vi "Cycle.vi"(8 "error in (no error)":errorcluster, 11 "MultDimExperiment In":refnum<class "MultDimExperiment.lvclass">) -> (0 "error out":errorcluster, 3 "MultDimExperiment Out":refnum<class "MultDimExperiment.lvclass">)   [LabVIEW 2010]
uses:
  MultDimExperiment.lvclass
panel:
  out "XY Graph":cluster{"horizontal":dbl[], "vertical":dbl[]}[](graph)
  out "ExperimentStats":T1
  in  "FixationRadius":dbl=50.0
  in  "RewardAmount":dbl=50.0
  in  "Timeouts":T2={"Intertrial"=1000.0, "AcquireFixation"=1000.0, "HoldFixation"=300.0, "DelayPeriod"=1000.0, "ResponsePeriod"=1000.0}
  in  "Eye Params":dbl[](array[numeric])
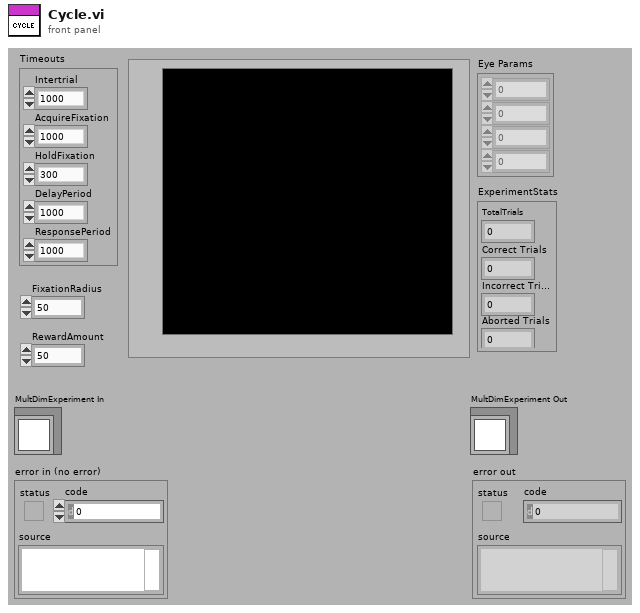
[diagram p1: front panel]
types:
  T1 = cluster{"TotalTrials":dbl, "Correct Trials":dbl, "Incorrect Trials":dbl, "Aborted Trials":dbl}
  T2 = cluster{"Intertrial":dbl, "AcquireFixation":dbl, "HoldFixation":dbl, "DelayPeriod":dbl, "ResponsePeriod":dbl}
  T3 = cluster{"TotalTrials":u32, "Correct Trials":u32, "Incorrect Trials":u32, "Aborted Trials":u32}
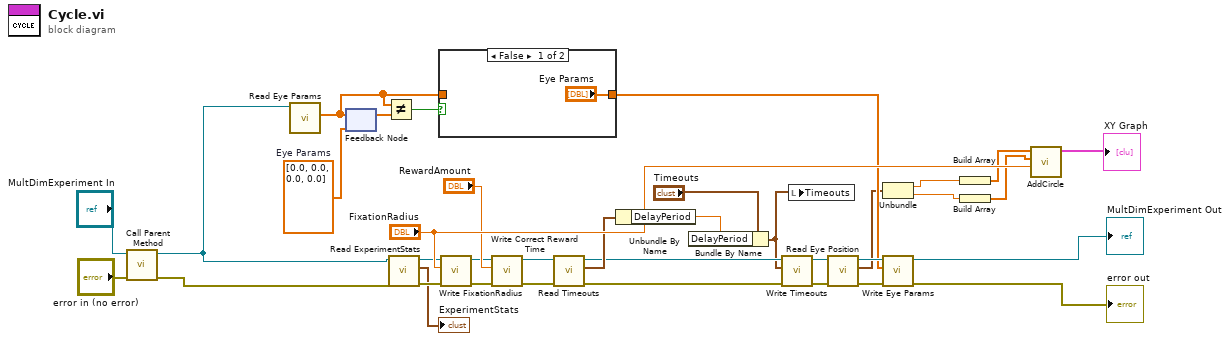
[diagram p0: block diagram]
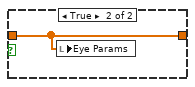
[diagram p2: hidden frame]
diagram:
  w17 = dbl[] [0.0, 0.0, 0.0, 0.0]  # Eye Params
  n1 = call-parent "Call Parent Method"("error in (no error)"="error in (no error)", "PassiveExperiment In"="MultDimExperiment In") -> ("error out"=w10:errorcluster, "PassiveExperiment Out"=w11:refnum<class "MultDimExperiment.lvclass">)  [unwired: 8 in]
  n2 = call-dynamic "Read Eye Params.vi"("TrialBasedExperiment in"=w11) -> ("Eye Params"=w16:dbl[])  [unwired: 8 in, 2 out]
  n3 = feedback #1(w17) -> (w19:dbl[])
  n4 = feedback-in #1(w16) -> ()
  n5 = Not Equal?(x=w16, y=w19) -> (x != y?=w18:bool)
  n6 = call-dynamic "Read ExperimentStats.vi"("error in (no error)"=w10, "TrialBasedExperiment in"=w11) -> ("error out"=w27:errorcluster, "ExperimentStats"=→"ExperimentStats":T3, "TrialBasedExperiment out"=w28:refnum<class "MultDimExperiment.lvclass">)  [unwired: 7 in]
  n7 = case shown="False" w18 {
    tunnel: ["Eye Params" w37] -> w13
    tunnel: w16 -> [_ w37]
    frame False {
    }
    frame True {
      n8 = local write "Eye Params"(w37) -> ()
    }
  }
  n9 = call-dynamic "Write FixationRadius.vi"("error in (no error)"=w27, "FixationRadius"="FixationRadius", "MatlabExperiment in"=w28) -> ("error out"=w24:errorcluster, "MatlabExperiment out"=w25:refnum<class "MultDimExperiment.lvclass">)  [unwired: 7 in]
  n10 = call-dynamic "Write Correct Reward Time.vi"("error in (no error)"=w24, "Correct Reward Time"="RewardAmount", "MatlabExperiment in"=w25) -> ("error out"=w22:errorcluster, "MatlabExperiment out"=w23:refnum<class "MultDimExperiment.lvclass">)  [unwired: 7 in]
  n11 = call-dynamic "Read Timeouts.vi"("error in (no error)"=w22, "TrialBasedExperiment in"=w23) -> ("error out"=w21:errorcluster, "Timeouts"=w6:T2, "TrialBasedExperiment out"=w5:refnum<class "MultDimExperiment.lvclass">)  [unwired: 7 in]
  n12 = Unbundle By Name(w6) -> ("DelayPeriod"=w7:dbl)
  n13 = Bundle By Name(cluster="Timeouts", "DelayPeriod"=w7) -> (w1:T2)
  n14 = call-dynamic "Write Timeouts.vi"("Timeouts"=w1, "TrialBasedExperiment in"=w5) -> ("TrialBasedExperiment out"=w3:refnum<class "MultDimExperiment.lvclass">)  [unwired: 8 in, 1 out]
  n15 = local write "Timeouts"(w1) -> ()
  n16 = call-dynamic "Read Eye Position.vi"("error in (no error)"=w21, "TrialBasedExperiment in"=w3) -> ("error out"=w14:errorcluster, "Eye Position"=w12:cluster{"Horizontal":dbl, "Vertical":dbl}, "TrialBasedExperiment out"=w15:refnum<class "MultDimExperiment.lvclass">)  [unwired: 7 in]
  n17 = Unbundle(w12) -> ("Horizontal"=w29:dbl, "Vertical"=w30:dbl)
  n18 = call-dynamic "Write Eye Params.vi"("error in (no error)"=w14, "Eye Params"=w13, "TrialBasedExperiment in"=w15) -> ("error out"=→"error out":errorcluster, "TrialBasedExperiment out"=→"MultDimExperiment Out":refnum<class "MultDimExperiment.lvclass">)  [unwired: 7 in]
  n19 = Build Array(w29) -> (w31:dbl[])
  n20 = Build Array(w30) -> (w32:dbl[])
  n21 = call "AddCircle.vi"("radius"="FixationRadius", "vertical"=w32, "horizontal"=w31) -> ("output"=→"XY Graph":cluster{"horizontal":dbl[], "vertical":dbl[]}[])  [unwired: 8 in]
